vi "Get Scheme.vi"(8 "error in (no error)":errorcluster, 11 "Protocol Config in":refnum<class "Protocol Config.lvclass">) -> (0 "error out":errorcluster, 2 "Scheme":string, 3 "Protocol Config out":refnum<class "Protocol Config.lvclass">)   [LabVIEW 2020, in "Examples.lvlib" / "Protocol Config.lvclass"]
uses:
  Protocol Config.lvclass
  Protocol Config.lvclass/Protocol Config.ctl
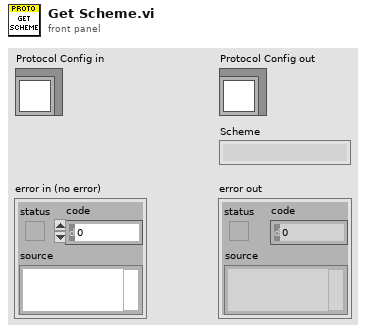
[diagram p1: front panel]
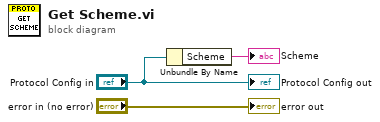
[diagram p0: block diagram]
diagram:
  n1 = Unbundle By Name("Protocol Config in") -> ("Scheme"=→"Scheme":string)
  "error out" <- "error in (no error)"
  "Protocol Config out" <- "Protocol Config in"
